vi "isNull.vi"(8 "error in (no error)":errorcluster, 11 "RealCustomer in":refnum<class "RealCustomer.lvclass">) -> (0 "error out":errorcluster, 2 "IsNull?":bool, 3 "RealCustomer out":refnum<class "RealCustomer.lvclass">)   [LabVIEW 2017, in "RealCustomer.lvclass"]
uses:
  RealCustomer.lvclass
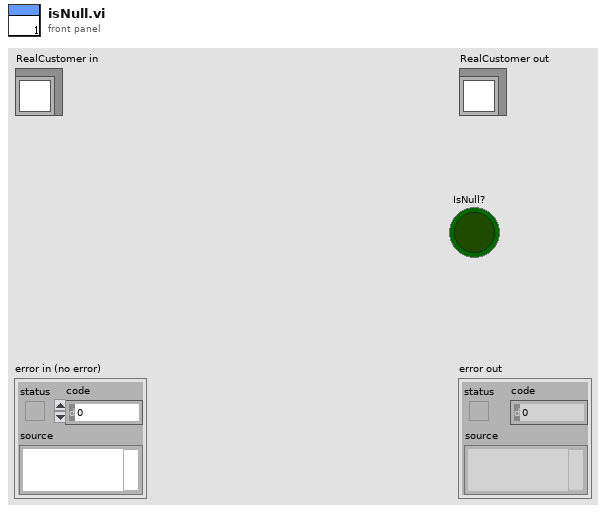
[diagram p1: front panel]
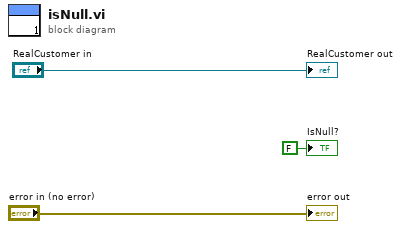
[diagram p0: block diagram]
diagram:
  "error out" <- "error in (no error)"
  "RealCustomer out" <- "RealCustomer in"
  "IsNull?" <- FALSE ("IsNull?")
